vi "Communicator_Create.vi"(8 "Error In":errorcluster, 11 "Communicator in":refnum<class "Communicator.lvclass">) -> (0 "Error Out":errorcluster, 3 "Communicator out":refnum<class "Communicator.lvclass">)   [LabVIEW 2024, in "Communicator.lvclass"]
uses:
  Communicator.lvclass
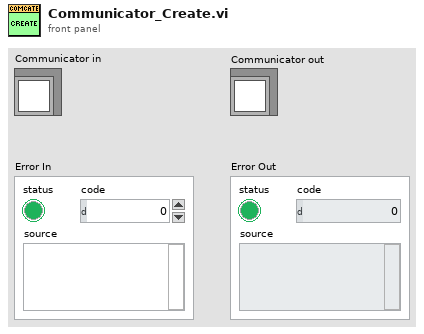
[diagram p1: front panel]
types:
  T1 = typedef "Communicator.lvclass/ObjectAttributes.ctl" = cluster{"IConfigure":refnum<class "IConfigure.lvclass">, "Worker Enqueuer":refnum<class "Message Enqueuer.lvclass">, "Start Counter":i32, "Msg Sent":refnum<user-event>}
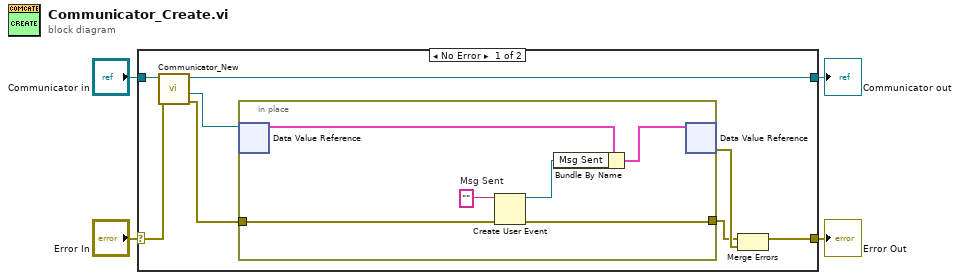
[diagram p0: block diagram]
diagram:
  n1 = case shown="No Error" "Error In" {
    selector: "Error In" -> [w11 w20]
    tunnel: [w7 w20] -> w3
    tunnel: "Communicator in" -> [w12 w19]
    tunnel: [w10 w19] -> w1
    frame No Error {
      n2 = call "Communicator_New.vi"("Error In"=w11, "Communicator in"=w12) -> ("Error Out"=w6:errorcluster, "DVRRefOut"=w8:refnum<data-value>, "Communicator out"=w10:refnum<class "Communicator.lvclass">)  [unwired: 6 in, 1 out]
      n3 = in-place {
        in-place-border: w6 -> [w15]
        in-place-border: [w14] -> w5
        w13 = ""  # Msg Sent
        n4 = in-place-dvr #1(w8) -> (w18:T1)  [unwired: 1 out]
        n5 = Create User Event(user event datatype=w13, error in=w15) -> (user event=w16:refnum<user-event>, error out=w14:errorcluster)
        n6 = Bundle By Name(cluster=w18, "Msg Sent"=w16) -> (w17:T1)
        n7 = in-place-dvr #1(w17) -> (w9:errorcluster)  [unwired: 1 out]
      }
      n8 = Merge Errors(w5, w9) -> (w7:errorcluster)
    }
    frame Error {
      # "VI-TechBaseTemplate_Simple_4x4x4"
    }
  }
  "Error Out" <- w3
  "Communicator out" <- w1
